vi "get_status.vi"(8 "error in (no error)":errorcluster, 11 "DS360 in":refnum<class "DS360.lvclass">) -> (0 "error out":errorcluster, 2 "status":cluster{"status":bool, "source":string}={"status"=TRUE, "source"=""}, 3 "DS360 out":refnum<class "DS360.lvclass">)   [LabVIEW 2019, in "DS360.lvclass"]
uses:
  DS360.lvclass
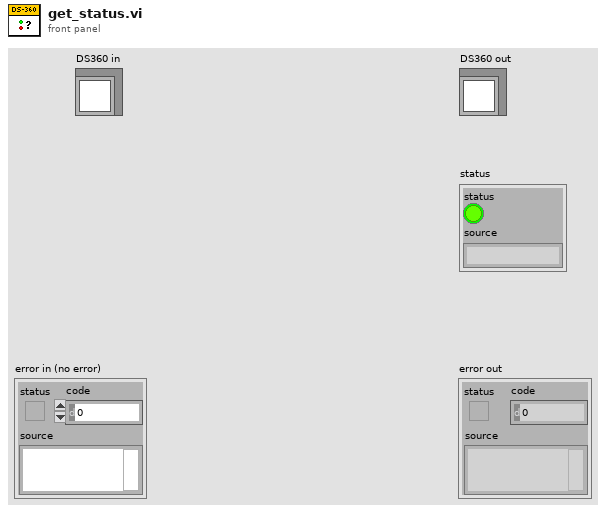
[diagram p1: front panel]
types:
  T1 = cluster{"error":bool, "code":i32, "source":string}
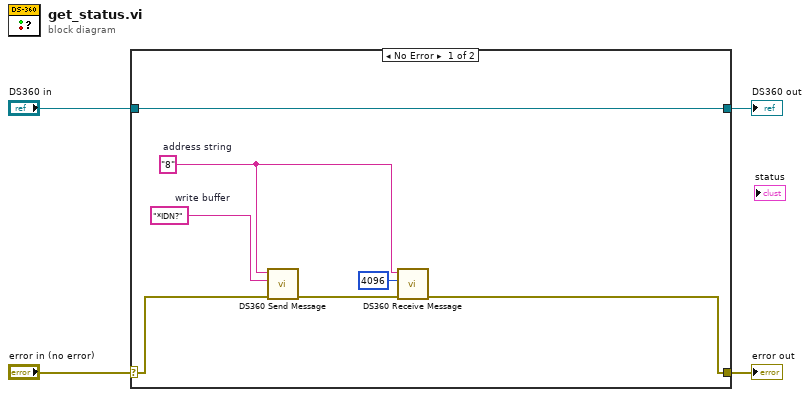
[diagram p0: block diagram]
diagram:
  n1 = case shown="No Error" "error in (no error)" {
    selector: "error in (no error)" -> [w6 w13]
    tunnel: [w5 w13] -> w3
    tunnel: [w11 w12] -> w1
    tunnel: "DS360 in" -> [w11 w12]
    frame No Error {
      w10 = "*IDN?"  # write buffer
      w8 = "8"  # address string
      n2 = call <instrlib>:"DS360 Send Message.vi"("address string"=w8, "write buffer"=w10, "error in"=w6) -> ("error out"=w9:T1)  [unwired: 3 in, 3 out]
      n3 = call <instrlib>:"DS360 Receive Message.vi"("address string"=w8, "byte count"=4096, "error in"=w9) -> ("error out"=w5:T1)  [unwired: 3 in, 3 out]
    }
    frame Error {
    }
  }
  "error out" <- w3
  "DS360 out" <- w1
